vi "String to V16__A2E.vi"(4 "Array of string Data":string[](array[string])) -> (1 "Array of V16":u16[](array[numeric]) format="%x")   [LabVIEW 2021, in "Strings.lvlib"]
doc: "This Vi convert a array of string in a array of V16 \n rules : each string is preceed by the number of characters follow-up by the ascii value of all of it. And all the blocks (Number+ascii code) are grouped and truncated in V16 array data.\nNote : if there is not enough characters a last 00 is add. \n\nThis convertion is usefull for typeDescriptor Data\n\nEric Bobillier INRA15/01/2007 France (eric.bobillier@rennes.inra.fr)"
uses:
  Strings/Strings.lvlib
panel:
  # "This Vi convert a array of string in a array of V16 \n rules : each string is preceed by the number of characters follow-up by the ascii value of all of it. \nAnd all the blocks (Number+ascii code) are grouped and truncated in V16 array data.\nNote : if there is not enough characters a last 00 is add. \n\nThis convertion is usefull for typeDescriptor Data\n\nEric Bobillier INRA15/01/2007  France   (eric.bobillier@rennes.inra.fr)"
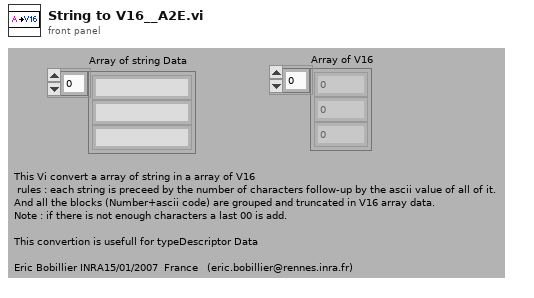
[diagram p1: front panel]
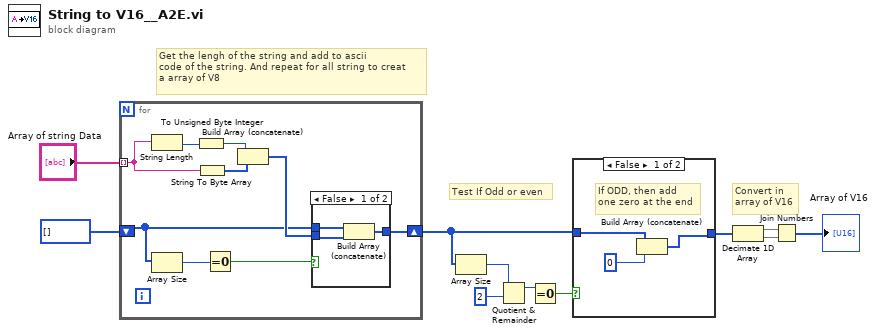
[diagram p0: block diagram]
diagram:
  # "Convert in \narray of V16"
  # "Test If Odd or even"
  # "Get the lengh of the string and add to ascii \ncode of the string. And repeat for all string to creat\na array of V8"
  n1 = for {
    tunnel: "Array of string Data" -> [w19] mode=indexing
    shift-right: [w15] -> w4
    shift-left: u8[] [] -> [w14]
    n2 = String Length(string=w19) -> (length=w20:i32)
    n3 = Array Size(array=w14) -> (size(s)=w13:i32)
    n4 = To Unsigned Byte Integer(number=w20) -> (unsigned 8bit integer=w18:u8)
    n5 = String To Byte Array(string=w19) -> (unsigned byte array=w17:u8[])
    n6 = Equal To 0?(x=w13) -> (x = 0?=w12:bool)
    n7 = Build Array (concatenate)(w18, w17) -> (w16:u8[])
    n8 = case shown="False" w12 {
      tunnel: w16 -> [w23 w24]
      tunnel: [w22 w24] -> w15
      tunnel: w14 -> [w21 _]
      frame False {
        n9 = Build Array (concatenate)(w21, w23) -> (w22:u8[])
      }
      frame True {
      }
    }
  }
  n10 = Array Size(array=w4) -> (size(s)=w8:i32)
  n11 = Quotient & Remainder(x=w8, y=2) -> (x-y*floor(x/y)=w5:i32)  [unwired: 1 out]
  n12 = Equal To 0?(x=w5) -> (x = 0?=w6:bool)
  n13 = case shown="False" w6 {
    tunnel: [w27 w28] -> w1
    tunnel: w4 -> [w25 w28]
    frame False {
      # "If ODD, then add \none zero at the end"
      n14 = Build Array (concatenate)(w25, u8 0) -> (w27:u8[])
    }
    frame True {
      # "Even Number of\nelements"
    }
  }
  n15 = Decimate 1D Array(w1) -> (w3:u8[], w2:u8[])
  n16 = Join Numbers(hi=w3, lo=w2) -> ((hi.lo)=→"Array of V16":u16[])
